vi "DAQ.vi"() -> ()   [LabVIEW 2025]
panel:
  out "Waveform Chart":dynamicdata(graph)
  in  "Stop Button":bool
  out "Temperature":dbl
  out "Thermometer":dbl(slide) scale=0.0..100.0
  # "LAB 2.2 DAQ-6009"
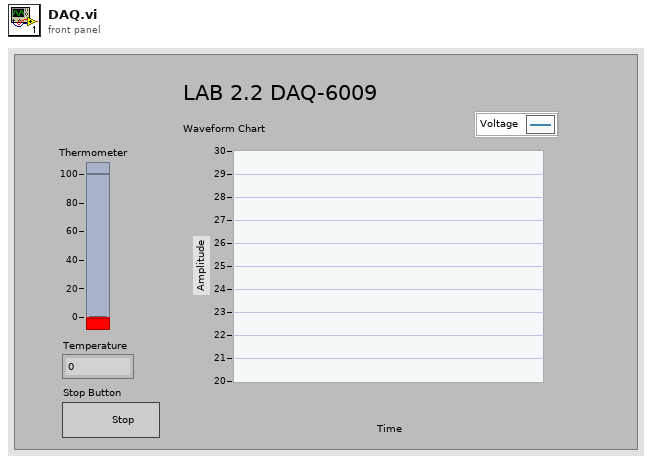
[diagram p1: front panel]
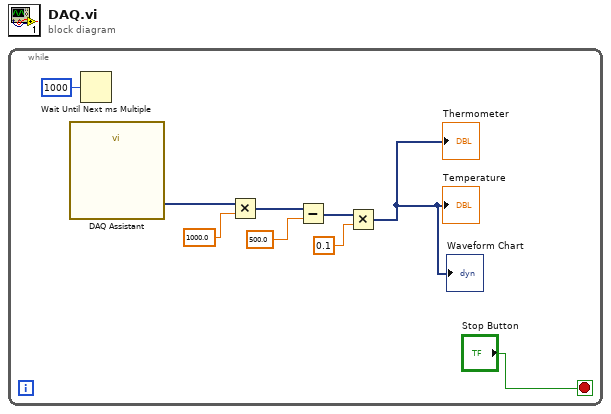
[diagram p0: block diagram]
diagram:
  n1 = while {
    stop <- "Stop Button" stop-if-true
    n2 = call "DAQ Assistant"() -> ("data"=w8:dynamicdata)  [unwired: 17 in, 2 out]
    n3 = Wait Until Next ms Multiple(millisecond multiple=u32 1000) -> ()  [unwired: 1 out]
    n4 = Multiply(x=w8, y=1000.0) -> (x*y=w6:dynamicdata)
    n5 = Subtract(x=w6, y=500.0) -> (x-y=w4:dynamicdata)
    n6 = Multiply(x=w4, y=0.1) -> (x*y=→"Thermometer" →"Temperature" →"Waveform Chart":dynamicdata)
  }
